vi "Reset.vi"(8 "error in (no error)":errorcluster, 11 "Proto Tag in":refnum<class "Basic Type.lvclass">) -> (0 "error out":errorcluster, 3 "Proto Tag out":refnum<class "Basic Type.lvclass">)   [LabVIEW 2020, in "Protobuf RAW.lvlib" / "Basic Type.lvclass"]
uses:
  Basic Type.lvclass
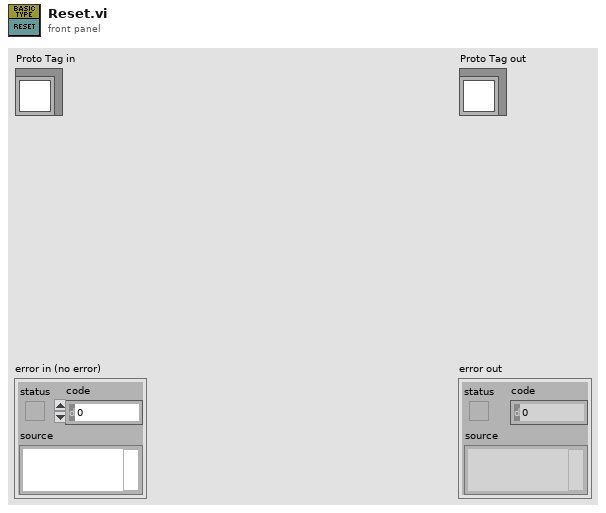
[diagram p1: front panel]
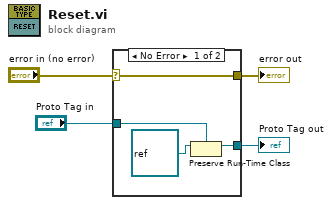
[diagram p0: block diagram]
diagram:
  n1 = case shown="No Error" "error in (no error)" {
    selector: "error in (no error)" -> [w7 w10]
    tunnel: [w7 w10] -> w3
    tunnel: [w6 w9] -> w1
    tunnel: "Proto Tag in" -> [w8 w9]
    frame No Error {
      n2 = Preserve Run-Time Class(object in=refnum<class> refnum, 2:w8) -> (object out=w6:refnum<class "Basic Type.lvclass">)  [unwired: 1 in, 1 out]
    }
    frame Error {
    }
  }
  "error out" <- w3
  "Proto Tag out" <- w1
